vi "ShowFP.vi"(8 "error in (no error)":errorcluster, 10 "ResetFP":bool caption="Reset Front Panel", 11 "CameraTestingUI in":refnum<class "CameraTestingUI.lvclass">) -> (0 "error out":errorcluster, 3 "CameraTestingUI out":refnum<class "CameraTestingUI.lvclass">)   [LabVIEW 2020, in "CameraTestingUI.lvlib" / "CameraTestingUI.lvclass"]
uses:
  CameraTestingUI.lvclass
  C:/Program Files (x86)/National Instruments/LabVIEW 2020/vi.lib/ActorFramework/Actor/Actor.lvclass
  CameraTestingUI.lvclass/CameraTestingUI.ctl
  <vilib>/ActorFramework/Actor/Actor.lvclass/Actor.ctl
  ICameraTesting/ICameraTesting Messages/LoadIntoSubPanel Msg/LoadIntoSubPanel Msg.lvclass/LoadIntoSubPanel Msg.ctl
  <vilib>/ActorFramework/Message Enqueuer/Message Enqueuer.lvclass/Message Enqueuer.ctl
  <vilib>/ActorFramework/Message Enqueuer/Enqueue.vi
  ICameraTesting/ICameraTesting Messages/LoadIntoSubPanel Msg/LoadIntoSubPanel Msg.lvclass
  C:/Program Files (x86)/National Instruments/LabVIEW 2020/vi.lib/ActorFramework/Message/Message.lvclass
  <vilib>/ActorFramework/Message Priority Queue/Priority Enqueue.vi
  <vilib>/ActorFramework/Actor/Actor.lvclass
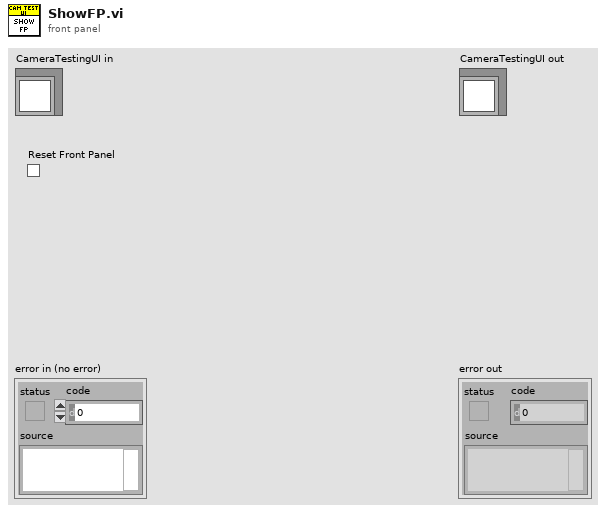
[diagram p1: front panel]
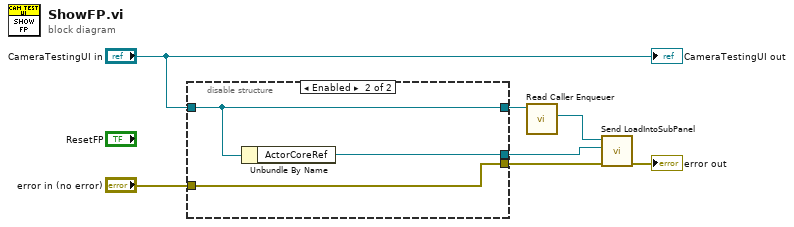
[diagram p0: block diagram]
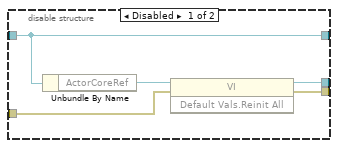
[diagram p2: hidden frame]
diagram:
  n1 = disable-structure shown="Enabled" {
    disable-tunnel: [w11 w13] -> w7
    disable-tunnel: "CameraTestingUI in" -> [w8 w15]
    disable-tunnel: [w10 w14] -> w4
    disable-tunnel: "error in (no error)" -> [w9 w13]
    disable-tunnel: [w8 w15] -> w1
    frame Disabled {
      n2 = Unbundle By Name(w8) -> ("ActorCoreRef"=w12:refnum<vi>)
      n3 = invoke class="VI" method="Default Vals.Reinit All"(reference=w12, error in=w9) -> (reference out=w10:refnum<vi>, error out=w11:errorcluster)  [unwired: 1 in, 1 out]
    }
    frame Enabled {
      n4 = Unbundle By Name(w15) -> ("ActorCoreRef"=w14:refnum<vi>)
    }
  }
  n5 = call <vilib>:"Read Caller Enqueuer.vi"("Actor"=w1) -> ("Caller Enqueuer"=w5:refnum<class "Message Enqueuer.lvclass">)  [unwired: 10 in]
  n6 = call "Send LoadIntoSubPanel.vi"("error in (no error)"=w7, "VI Refnum"=w4, "Message Enqueuer"=w5) -> ("error out"=→"error out":errorcluster)  [unwired: 7 in, 1 out]
  "CameraTestingUI out" <- "CameraTestingUI in"
